vi "FuncImg-Reset panes.vi"   [LabVIEW 2020]
uses:
  <vilib>/Utility/miscctls.llb/LVPointTypeDef.ctl
  Global variables/gl_Functional Imaging-Global variables.vi
types:
  T1 = typedef "LVPointTypeDef.ctl" = cluster{"Horizontal":i16, "Vertical":i16}
  T2 = typedef "Functional Imging UI Refs.ctl" = cluster{"Menu ref":refnum<k9>, "Image control":refnum<vi>, "VI ref":refnum<vi>, "XGrapher":refnum<vi>, "Smoothing":refnum<vi>, "POI Averaging":refnum<vi>, "Normalize":refnum<vi>, "POI data points in each trial":refnum<vi>, "Channel":refnum<vi>, "Experiment data folder path":refnum<vi>, "[ROI vis]":refnum<vi>, "[Groups] visbl":T3, "Group Name":refnum<vi>, "POI index":refnum<vi>, "Trial No.":refnum<vi>, "Intensity Zoom":refnum<vi>, "Trial Cursor Enabled":refnum<vi>, "Number of Trials (ind 1)":refnum<vi>, "Number of Trials (ind 2)":refnum<vi>, "MiniScans Available":refnum<vi>, "POI Available":refnum<vi>, "Defer graph updates":refnum<vi>, "Waveform selector":refnum<vi>, "#of selected POI":refnum<vi>, "#of selected MiniScans":refnum<vi>, "#of selected groups":refnum<vi>, "Max Z-Projection":refnum<vi>, "Z-Plane Selector":refnum<vi>, "Index of miniscan point to visualise":refnum<vi>, "ROI vis. mode":refnum<vi>, "Total # of points":refnum<vi>, "Index of group clicked on":refnum<vi>, "Pane 1":refnum<vi>, "Pane 2":refnum<vi>, "Pane 3":refnum<vi>, "Pane 4":refnum<vi>, "Pane 5":refnum<vi>, "Pane 6":refnum<vi>, "Deselect all ROI":refnum<vi>, "Deselect all groups":refnum<vi>}
  T3 = typedef "Groups array referecne.ctl" = refnum<vi>
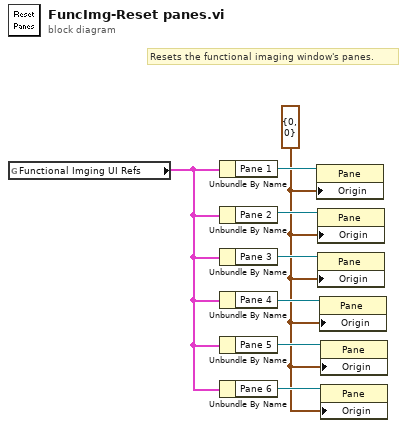
[diagram p0: block diagram]
diagram:
  w1 = T1 {"Horizontal"=0, "Vertical"=0} ("Origin")
  # "Resets the functional imaging window's panes."
  n1 = global read "gl_Functional Imaging-Global variables.vi" "Functional Imging UI Refs"() -> (w8:T2)
  n2 = Unbundle By Name(w8) -> ("Pane 1"=w2:refnum<vi>)
  n3 = Unbundle By Name(w8) -> ("Pane 2"=w3:refnum<vi>)
  n4 = Unbundle By Name(w8) -> ("Pane 3"=w4:refnum<vi>)
  n5 = Unbundle By Name(w8) -> ("Pane 4"=w5:refnum<vi>)
  n6 = Unbundle By Name(w8) -> ("Pane 5"=w6:refnum<vi>)
  n7 = Unbundle By Name(w8) -> ("Pane 6"=w7:refnum<vi>)
  n8 = property on="Property Node" class="Pane"(reference=w2, "Origin"=w1) -> ()  [unwired: 1 in, 2 out]
  n9 = property on="Property Node" class="Pane"(reference=w3, "Origin"=w1) -> ()  [unwired: 1 in, 2 out]
  n10 = property on="Property Node" class="Pane"(reference=w4, "Origin"=w1) -> ()  [unwired: 1 in, 2 out]
  n11 = property on="Property Node" class="Pane"(reference=w5, "Origin"=w1) -> ()  [unwired: 1 in, 2 out]
  n12 = property on="Property Node" class="Pane"(reference=w6, "Origin"=w1) -> ()  [unwired: 1 in, 2 out]
  n13 = property on="Property Node" class="Pane"(reference=w7, "Origin"=w1) -> ()  [unwired: 1 in, 2 out]
